vi "Get Limits.vi"(0 "reference in":refnum<class "Simulated-PowerModule.lvclass">, 11 "Error In":errorcluster) -> (4 "reference out":refnum<class "Simulated-PowerModule.lvclass">, 6 "Limits":T1, 15 "Error Out":errorcluster)   [LabVIEW 2023, in "Simulated-PowerModule.lvlib" / "Simulated-PowerModule.lvclass"]
uses:
  Simulated-PowerModule.lvclass
  builds/PowerModuleInterface/home/lvuser/natinst/bin/PowerModuleInterface.lvlibp/Classes/PowerModule_interface/Limits.ctl
  builds/PowerModuleInterface/home/lvuser/natinst/bin/PowerModuleInterface.lvlibp/Classes/PowerModule_interface/PowerModuleInterface.lvclass
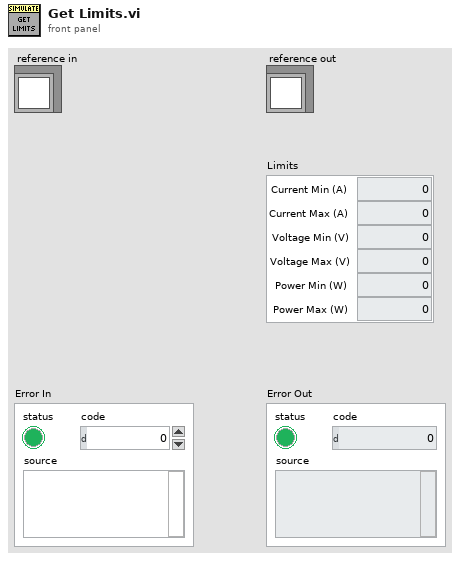
[diagram p1: front panel]
types:
  T1 = typedef "PowerModuleInterface.lvlibp/PowerModuleInterface.lvclass/Limits.ctl" = cluster{"Current Max (A)":dbl, "Current Min (A)":dbl, "Voltage Max (V)":dbl, "Voltage Min (V)":dbl, "Power Max (W)":dbl, "Power Min (W)":dbl}
  T2 = typedef "Simulated-PowerModule.lvlib/Simulated-PowerModule.lvclass/ObjectAttributes.ctl" = cluster{"JSON Config Path":path, "Configuration":T3, "connected":bool, "reserved":bool, "energized":bool, "output enabled":bool, "Mode":T4, "Range":T5, "Slew Rates":T6, "Setpoints":cluster{"voltage":dbl, "current":dbl, "resistance":dbl}, "Measurements":cluster{"voltage":dbl, "current":dbl, "resistance":dbl}, "Limits":T1, "active faults":string[], "fault":bool, "profile":dbl[][], "step dt":i64}
  T3 = typedef "Simulated-PowerModule.lvlib/Simulated-PowerModule.lvclass/Configuration.ctl" = cluster{"IP Address":string}
  T4 = typedef "Simulated-PowerModule.lvlib/Simulated-PowerModule.lvclass/Mode.ctl" = u16
  T5 = typedef "PowerModuleInterface.lvlibp/PowerModuleInterface.lvclass/Range.ctl" = cluster{"Current Max (A)":dbl, "Current Min (A)":dbl, "Voltage Max (V)":dbl, "Voltage Min (V)":dbl}
  T6 = typedef "PowerModuleInterface.lvlibp/PowerModuleInterface.lvclass/Slew Rates.ctl" = cluster{"Current Decrease (A/sec)":dbl, "Current Increase (A/sec)":dbl, "Voltage Decrease (V/sec)":dbl, "Voltage Increase (V/sec)":dbl, "Resistance Decrease (Ohm/sec)":dbl, "Resistance Increase (Ohm/sec)":dbl}
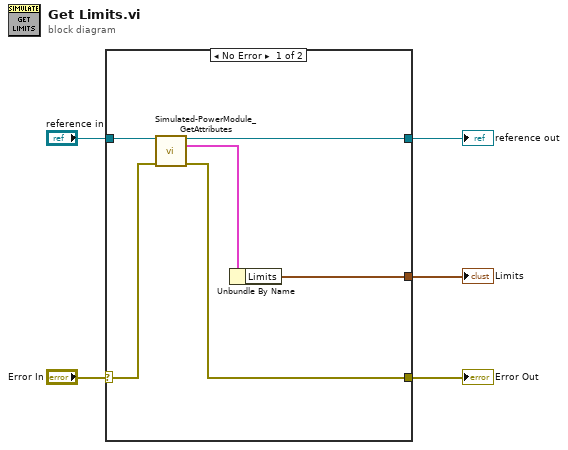
[diagram p0: block diagram]
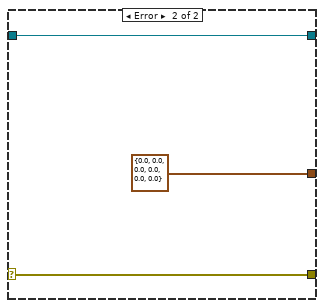
[diagram p2: hidden frame]
diagram:
  n1 = case shown="No Error" "Error In" {
    selector: "Error In" -> [w10 w13]
    tunnel: "reference in" -> [w11 w14]
    tunnel: [w9 w14] -> w4
    tunnel: [w8 w13] -> w2
    tunnel: [w6 T1 {"Current Max (A)"=0.0, "Current Min (A)"=0.0, "Voltage Max (V)"=0.0, "Voltage Min (V)"=0.0, "Power Max (W)"=0.0, "Power Min (W)"=0.0} ("Limits")] -> w1
    frame No Error {
      n2 = call "Simulated-PowerModule_GetAttributes.vi"("reference in"=w11, "Error In"=w10) -> ("reference out"=w9:refnum<class "Simulated-PowerModule.lvclass">, "Data"=w7:T2, "Error Out"=w8:errorcluster)  [unwired: 10 in, 1 out]
      n3 = Unbundle By Name(w7) -> ("Limits"=w6:T1)
    }
    frame Error {
    }
  }
  "Error Out" <- w2
  "reference out" <- w4
  "Limits" <- w1
